vi "[PC]LogGlobVar.vi"() -> ()   [LabVIEW 2018]
uses:
  RT/[GlobVar]SensorState.vi
panel:
  out "Datasets Logged":i32
  out "LogFileRef":refnum<k34>
  out "LogFilePath":path
  out "LogfileName":string
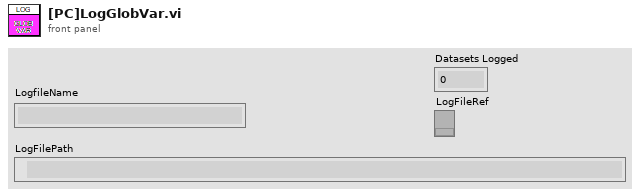
[diagram p1: front panel]
types:
  T1 = enum16{"open", "open or create", "create or replace", "create", "open (read-only)"}
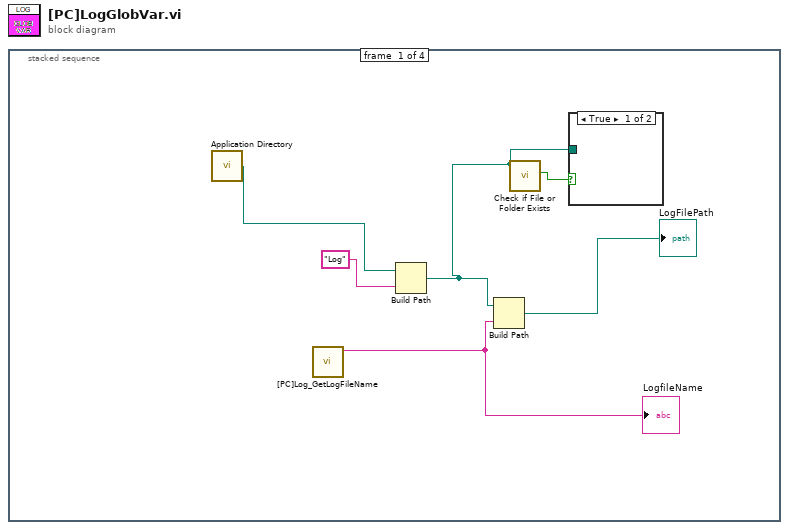
[diagram p0: block diagram]
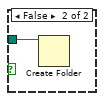
[diagram p2: hidden frame]
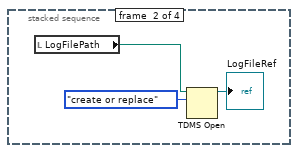
[diagram p3: hidden frame]
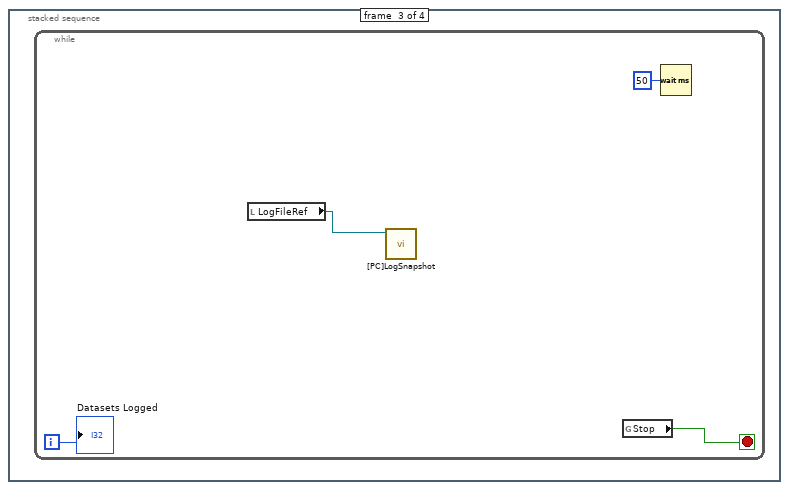
[diagram p4: hidden frame]
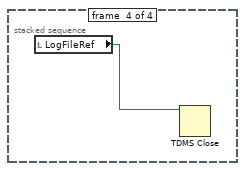
[diagram p5: hidden frame]
diagram:
  n1 = stacked-sequence {
    frame #0 {
      n2 = call <vilib>:"Application Directory.vi"() -> ("Application Directory"=w4:path)
      n3 = call "[PC]Log_GetLogFileName.vi"() -> ("String"=w5:string)  [unwired: 11 in]
      "LogfileName" <- w5
      n4 = Build Path(base path=w4, name or relative path="Log") -> (appended path=w2:path)
      n5 = Build Path(base path=w2, name or relative path=w5) -> (appended path=→"LogFilePath":path)
      n6 = call <vilib>:"Check if File or Folder Exists.vi"("path"=w2) -> ("file or folder exists?"=w1:bool)  [unwired: 8 in, 2 out]
      n7 = case shown="True" w1 {
        tunnel: w2 -> [_ w7]
        frame True {
        }
        frame False {
          n8 = Create Folder(path (use dialog)=w7) -> ()  [unwired: 2 in, 3 out]
        }
      }
    }
    frame #1 {
      n9 = local read "LogFilePath"() -> (w8:path)
      n10 = TDMS Open(10:T1."create or replace" ("Operation (0:Öffnen)"), 11:w8) -> (3:→"LogFileRef":refnum<k34>)  [unwired: 5 in, 1 out]
    }
    frame #2 {
      n11 = while {
        i -> [w12]
        stop <- w14 stop-if-true
        n12 = local read "LogFileRef"() -> (w11:refnum<k34>)
        n13 = call "[PC]LogSnapshot.vi"("LogFileRef"=w11) -> ()  [unwired: 11 in]
        n14 = global read "[GlobVar]SensorState.vi" "Stop"() -> (w14:bool)
        n15 = Wait (ms)(milliseconds to wait=u32 50) -> ()  [unwired: 1 out]
        "Datasets Logged" <- w12
      }
    }
    frame #3 {
      n16 = local read "LogFileRef"() -> (w15:refnum<k34>)
      n17 = TDMS Close(11:w15) -> ()  [unwired: 1 in, 2 out]
    }
  }
